vi "Periodic Tasks.vi"(8 "error in":errorcluster) -> ()   [LabVIEW 2016]
doc: "This VI runs in parallel to other tasks. It can contain as many user-defined periodic loops as you need. These can carry out PID or other sorts of timed response."
uses:
  <vilib>/Rock Robotics/WPI/Utilities/WPI_GetSetVariantRefNum.vi
  test2/Robot Global Data.vi
  <vilib>/Rock Robotics/WPI/RobotDrive/WPI_RobotDriveArcadeDrive_Standard(NoSaturation).vi
  <vilib>/Rock Robotics/Network Tables/NT Write Number.vi
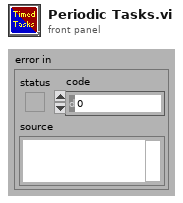
[diagram p1: front panel]
types:
  T1 = typedef "WPI_RobotDriveDevRef.ctl" = cluster{"DevStatus":errorcluster, "Motors[]":T2[], "Square Inputs":bool, "Max Output":dbl}
  T2 = typedef "WPI_MotorControlDeviceRef.ctl" = cluster{"DeviceStatus":errorcluster, "Type":T3, "PWM":cluster{"PWM Channel":T4, "DeadBand":T5}, "CAN":cluster{"Device Number":u8, "SetOutput VI Ref":variant, "GetOutput VI Ref":variant, "Enable VI Ref":variant, "Disable VI Ref":variant, "Data":variant}, "Invert":bool}
  T3 = typedef "WPI_MotorControlType.ctl" = enum16{"PWM", "CAN"}
  T4 = typedef "FPGA_DIOPWMChannel.ctl" = enum8{"PWM 0", "PWM 1", "PWM 2", "PWM 3", "PWM 4", "PWM 5", "PWM 6", "PWM 7", "PWM 8", "PWM 9", "PWM MXP 0", "PWM MXP 1", "PWM MXP 2", "PWM MXP 3", "PWM MXP 4", "PWM MXP 5", "PWM MXP 6", "PWM MXP 7", "PWM MXP 8", "PWM MXP 9", "Invalid"}
  T5 = typedef "WPI_PWMDeadband.ctl" = cluster{"Name":string, "maxPositivePwm":i32, "minPositivePwm":i32, "centerPwm":i32, "maxNegativePwm":i32, "minNegativePwm":i32, "angularRange":u16}
  T6 = typedef "WPI_JoystickDevRef.ctl" = cluster{"Device":T7}
  T7 = typedef "WPI_JoystickDeviceEnum.ctl" = enum16{"USB 0", "USB 1", "USB 2", "USB 3", "USB 4", "USB 5"}
  T8 = typedef "WPI_EncoderDevRef.ctl" = cluster{"DevStatus":errorcluster, "EncoderIndex":T9, "CounterIndex":T10, "DistancePerCount":dbl, "Decoding Type":T11}
  T9 = typedef "FPGA_EncoderIdx.ctl" = enum8{"Enc 0", "Enc 1", "Enc 2", "Enc 3", "Enc 4", "Enc 5", "Enc 6", "Enc 7", "Invalid"}
  T10 = typedef "FPGA_CounterCtrSystemIndex.ctl" = enum8{"Ctr 0", "Ctr 1", "Ctr 2", "Ctr 3", "Ctr 4", "Ctr 5", "Ctr 6", "Ctr 7", "Invalid"}
  T11 = typedef "WPI_EncoderType.ctl" = enum16{"1x", "2x", "4x"}
  T12 = cluster{"JoystickDevRef":T6, "RobotDriveDevRef":T1}
  T13 = typedef "WPI_DriverStationRobotMode2.ctl" = enum16{"Autonomous Disabled", "Autonomous Enabled", "Teleop Disabled", "Teleop Enabled", "Disconnected", "Finish", "Test Disabled", "Test Enabled", "Emergency Stopped"}
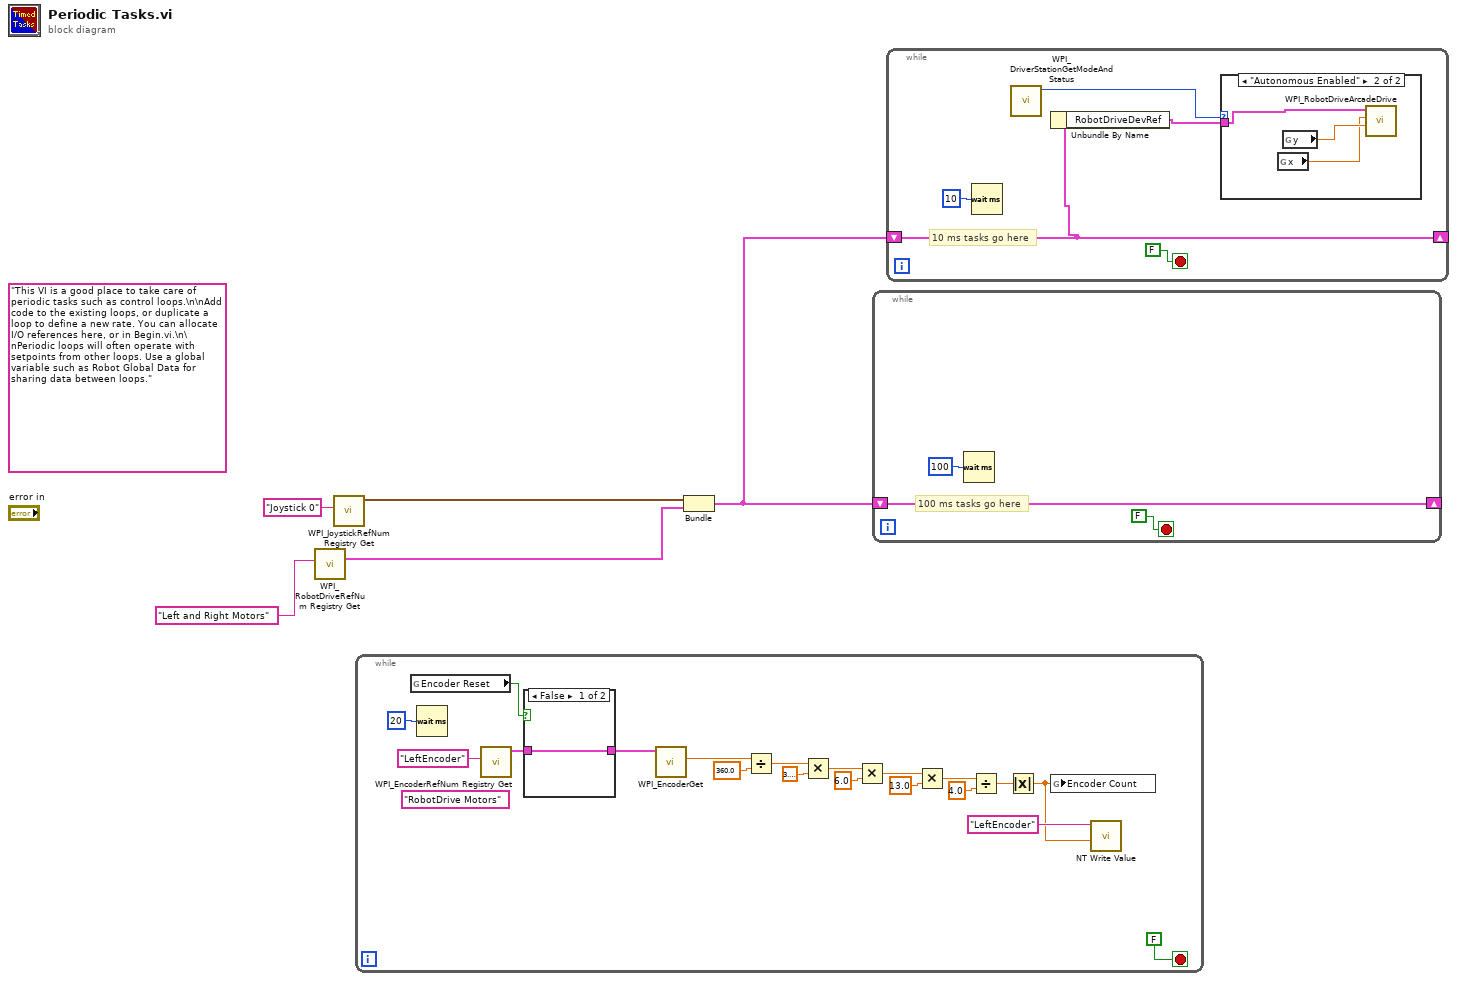
[diagram p0: block diagram]
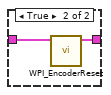
[diagram p2: hidden frame]
diagram:
  (unwired) "This VI is a good place to take care of periodic tasks such as control loops.\n\nAdd code to the existing loops, or duplicate a loop to define a new rate. You can allocate I/O references here, or in Begin.vi.\n\nPeriodic loops will often operate with setpoints from other loops. Use a global variable such as Robot Global Data for sharing data between loops."
  n1 = call <vilib>:"WPI_RobotDriveRefNum Registry Get.vi"("refnum name"="Left and Right Motors") -> ("RobotDriveDevRef"=w1:T1)  [unwired: 1 in, 9 out]
  n2 = call <vilib>:"WPI_JoystickRefNum Registry Get.vi"("refnum name"="Joystick 0") -> ("JoystickDevRef"=w3:T6)  [unwired: 1 in, 9 out]
  n3 = while {
    stop <- FALSE stop-if-true
    (unwired) "RobotDrive Motors" ("Name")
    n4 = global read "Robot Global Data.vi" "Encoder Reset"() -> (w11:bool)
    n5 = Wait (ms)(milliseconds to wait=u32 20) -> ()  [unwired: 1 out]
    n6 = call <vilib>:"WPI_EncoderRefNum Registry Get.vi"("refnum name"="LeftEncoder") -> ("EncoderDevRef"=w10:T8)  [unwired: 9 in, 1 out]
    n7 = case shown="False" w11 {
      tunnel: [w25 w27] -> w9
      tunnel: w10 -> [w25 w26]
      frame False {
      }
      frame True {
        n8 = call <vilib>:"WPI_EncoderReset.vi"("EncoderDevRef"=w26) -> ("EncoderDevRef"=w27:T8)  [unwired: 9 in, 1 out]
      }
    }
    n9 = call <vilib>:"WPI_EncoderGet.vi"("EncoderDevRef"=w9) -> ("Distance"=w13:dbl)  [unwired: 5 in, 5 out]
    n10 = Divide(x=w13, y=360.0) -> (x/y=w19:dbl)
    n11 = Multiply(x=w19, y=3.141592653589793) -> (x*y=w22:dbl)
    n12 = Multiply(x=w22, y=6.0) -> (x*y=w14:dbl)
    n13 = Multiply(x=w14, y=13.0) -> (x*y=w15:dbl)
    n14 = Divide(x=w15, y=4.0) -> (x/y=w7:dbl)
    n15 = Absolute Value(x=w7) -> (abs(x)=w6:dbl)
    n16 = global write "Robot Global Data.vi" "Encoder Count"(w6) -> ()
    n17 = call-poly <vilib>:"NT Write Value.vi"("Numeric"=w6, "Name"="LeftEncoder") -> ()  [unwired: 9 in, 1 out]
  }
  n18 = Bundle("JoystickDevRef"=w3, "RobotDriveDevRef"=w1) -> (w2:T12)  [unwired: 1 out]
  n19 = while {
    shift-right: [w28] -> _
    shift-left: w2 -> [w28]
    stop <- FALSE stop-if-true
    # "100 ms tasks go here"
    n20 = Wait (ms)(milliseconds to wait=u32 100) -> ()  [unwired: 1 out]
  }
  n21 = while {
    shift-right: [w31] -> _
    shift-left: w2 -> [w31]
    stop <- FALSE stop-if-true
    # "10 ms tasks go here"
    n22 = Wait (ms)(milliseconds to wait=u32 10) -> ()  [unwired: 1 out]
    n23 = call <vilib>:"WPI_DriverStationGetModeAndStatus.vi"() -> ("Robot Mode"=w32:T13)  [unwired: 10 in, 1 out]
    n24 = Unbundle By Name(w31) -> ("RobotDriveDevRef"=w33:T1)
    n25 = case shown="\"Autonomous Enabled\"" w32 {
      tunnel: w33 -> [_ w38]
      frame "Autonomous Disabled", Default {
      }
      frame "Autonomous Enabled" {
        n26 = global read "Robot Global Data.vi" "x"() -> (w36:dbl)
        n27 = global read "Robot Global Data.vi" "y"() -> (w37:dbl)
        n28 = call-poly <vilib>:"WPI_RobotDriveArcadeDrive.vi"("Y axis value"=w37, "X axis value"=w36, "RobotDriveDevRef"=w38) -> ()  [unwired: 6 in, 3 out]
      }
    }
  }
